vi "Save Controls Attribute.vi"(8 "error in (no error)":errorcluster, 10 "Control Refs":refnum<vi>[](array[refnum]), 11 "ScriptSettingConfiguration in":refnum<class "ScriptSettingConfiguration.lvclass">) -> (0 "error out":errorcluster, 3 "ScriptSettingConfiguration out":refnum<class "ScriptSettingConfiguration.lvclass">)   [LabVIEW 2015, in "ScriptSettingConfiguration.lvclass"]
uses:
  ScriptSettingConfiguration.lvclass
  UIConfiguration/UIConfiguration.lvclass
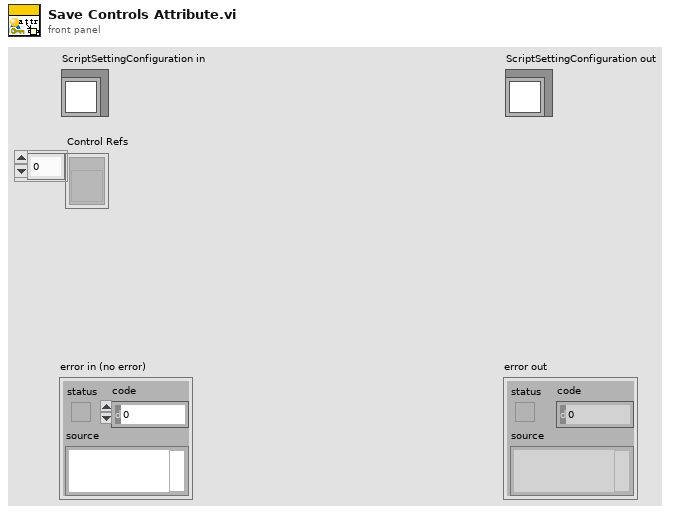
[diagram p1: front panel]
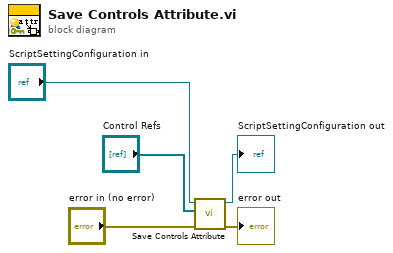
[diagram p0: block diagram]
diagram:
  n1 = call-parent "Save Controls Attribute.vi"("error in (no error)"="error in (no error)", "Control Refs"="Control Refs", "UIConfiguration in"="ScriptSettingConfiguration in") -> ("error out"=→"error out":errorcluster, "UIConfiguration out"=→"ScriptSettingConfiguration out":refnum<class "ScriptSettingConfiguration.lvclass">)  [unwired: 7 in]
